vi "SVT Fractional-octave Analysis.vi"   [LabVIEW 2017, in "SoundVib_Octave_2014 standard.lvlib"]
doc: "Performs a fractional-octave analysis on <B>scaled signal [EU]</B> in accordance with the IEC 61260:2014 and ANSI S1.11-2014 standards. Wire data to the <B>scaled signal [EU]</B> input to determine the polymorphic instance to use or manually select the instance."
uses:
  <vilib>/addons/Sound and Vibration/svt_Octave/SoundVib_Octave_2014 standard.lvlib
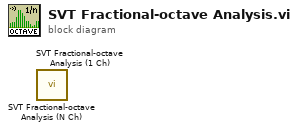
[diagram p0: block diagram]
diagram:
  n1 = call <vilib>:"SVT Fractional-octave Analysis (N Ch).vi"() -> ()  [unwired: 10 in, 6 out]
  n2 = call <vilib>:"SVT Fractional-octave Analysis (1 Ch).vi"() -> ()  [unwired: 10 in, 6 out]
